vi "Add State(s) to Queue By BOOL(Array Right).vi"(4 "False(Empty)":string[](array[string]), 6 "TRUE(Empty)":string, 8 "High Priority(FALSE)":bool, 10 "Bool":bool, 11 "Remaining States":string) -> (3 "States Out":string)   [LabVIEW 2014, in "JKI-State-Machine-Plus.lvlib"]
doc: "Depending on the High Priority and Bool input, this VI generates a concatenated state of TRUE/False and Remaning States. The High Priority input determines if the TRUE or False string concatenates before/after the remaining states. The Bool input determines whether TRUE or False string to be concatenated."
uses:
  JKI-State-Machine-Plus.lvlib
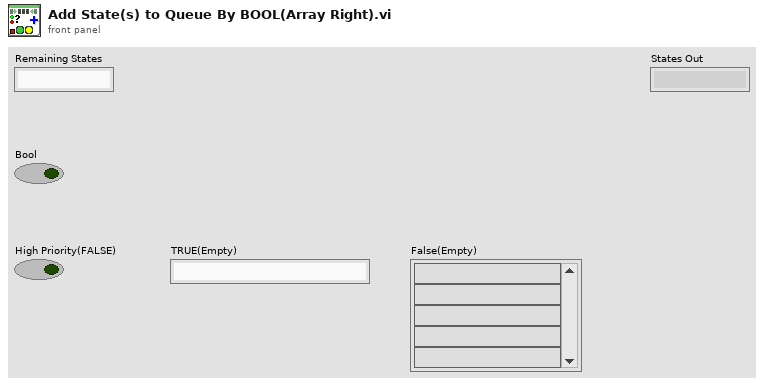
[diagram p1: front panel]
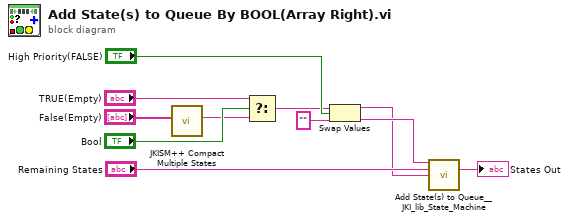
[diagram p0: block diagram]
diagram:
  n1 = call "JKISM++ Compact Multiple States.vi"("States in Lines"="False(Empty)") -> ("States"=w1:string)  [unwired: 9 in]
  n2 = Select(t="TRUE(Empty)", s="Bool", f=w1) -> (s? t:f=w5:string)
  n3 = Swap Values(12:w5, 13:"High Priority(FALSE)", 14:"") -> (1:w2:string, 3:w3:string)
  n4 = call <vilib>:"Add State(s) to Queue__JKI_lib_State_Machine.vi"("State(s) in Front (\"\")"=w3, "State(s) in (\"\")"="Remaining States", "State(s) at Back (\"\")"=w2) -> ("States Out"=→"States Out":string)  [unwired: 12 in]
